vi "GetAllAMC.vi"(7 "LabVIEW Web Service Request":refnum<class "Web Request.lvclass">) -> ()   [LabVIEW 2021]
uses:
  <vilib>/wsapi/Web Request.lvclass
  <vilib>/addons/database/NI_Database_API.lvlib
  <vilib>/addons/database/Connection.llb/Conn Execute.vi
  <vilib>/addons/database/Recordset.llb/Rec Fetch Recordset Data (R).vi
  <vilib>/addons/database/Connection.llb/DB Tools Open Connec (Path).vi
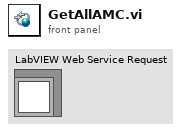
[diagram p1: front panel]
types:
  T1 = typedef "NI_Database_API.lvlib/Conn ObjectReference.ctl" = refnum<k1>
  T2 = typedef "NI_Database_API.lvlib/Rec ObjectReference.ctl" = refnum<k1>
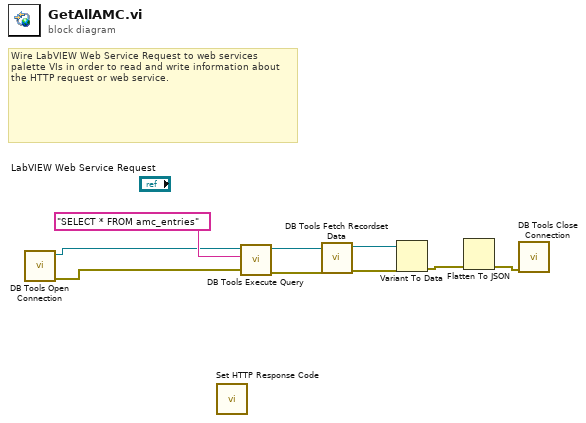
[diagram p0: block diagram]
diagram:
  # "Wire LabVIEW Web Service Request to web services palette VIs in order to read and write information about the HTTP request or web service."
  n1 = call-poly <vilib>:"DB Tools Open Connection.vi"() -> ("error out"=w6:errorcluster, "connection reference"=w8:T1)  [unwired: 8 in]
  n2 = call <vilib>:"Set HTTP Response Code.vi"() -> ()  [unwired: 14 in, 2 out]
  n3 = call-poly <vilib>:"DB Tools Execute Query.vi"("error in (no error)"=w6, "SQL query"="SELECT * FROM amc_entries", "connection reference"=w8) -> ("error out"=w5:errorcluster, "recordset reference"=w7:T2)  [unwired: 5 in]
  n4 = call-poly <vilib>:"DB Tools Fetch Recordset Data.vi"("error in (no error)"=w5, "recordset reference"=w7) -> ("error out"=w4:errorcluster, "recordset reference out"=w1:T2)  [unwired: 3 in, 1 out]
  n5 = Variant To Data(error in=w4, Variant=w1) -> (error out=w3:errorcluster)  [unwired: 1 in, 1 out]
  n6 = Flatten To JSON(error in (no error)=w3) -> (11:w2:errorcluster)  [unwired: 2 in, 1 out]
  n7 = call <vilib>:"DB Tools Close Connection.vi"("error in (no error)"=w2) -> ()  [unwired: 6 in, 1 out]
